vi "QueryServer_CreateServer.vi"() -> (3 "gRPCid":T1)   [LabVIEW 2019, in "labview-grpc-query-server.lvlib"]
uses:
  labview-grpc-query-server.lvlib
  QueryServer_gRPCid.ctl
  build/Debug/labview_query_server.dll
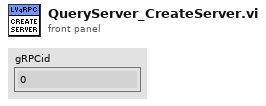
[diagram p1: front panel]
types:
  T1 = typedef "labview-grpc-query-server.lvlib/QueryServer_gRPCid.ctl" = u64
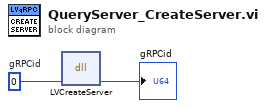
[diagram p0: block diagram]
diagram:
  w2 = T1 0  # gRPCid
  n1 = dll-call lib="C:/dev/labview-grpc-query-server/build/Debug/labview_query_server.dll" fn="LVCreateServer"(w2) -> (→"gRPCid":T1)  [unwired: 4 in, 2 out]
